vi "Polar (SubVI).vi"(11 "priorCoord":cluster{"x prior ":i32, "y prior":i32}) -> (2 "magnitude":dbl format="%0.2f", 3 "phase":dbl)   [LabVIEW 2011]
uses:
  <vilib>/Analysis/coordinate.llb/Angle Range (Degree).ctl
  <vilib>/Analysis/coordinate.llb/Angle Units.ctl
  <vilib>/Analysis/coordinate.llb/Wrap Angle (scalar).vi
  <vilib>/Analysis/NI_AAL_Angle.lvlib
  <vilib>/ptbypt/NI_PtbyPt.lvlib
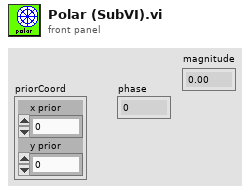
[diagram p1: front panel]
types:
  T1 = typedef "NI_AAL_Angle.lvlib/Angle Units.ctl" = i32
  T2 = typedef "NI_AAL_Angle.lvlib/Angle Range (Degree).ctl" = u16
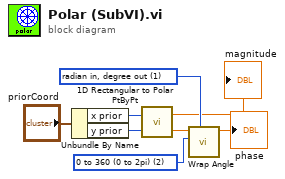
[diagram p0: block diagram]
diagram:
  w6 = T1 1 items=["radian in, radian out", "radian in, degree out", "degree in, degree out", "degree in, radian out"] ("angle units")
  w5 = T2 2 items=["none", "-180 to 180 (-pi to pi)", "0 to 360 (0 to 2pi)"] ("angle range")
  n1 = Unbundle By Name("priorCoord") -> ("x prior"=w2:i32, "y prior"=w3:i32)
  n2 = call <vilib>:"1D Rectangular to Polar PtByPt.vi"("y"=w3, "x"=w2) -> ("phase"=w4:dbl, "magnitude"=→"magnitude":dbl)
  n3 = call-poly <vilib>:"Wrap Angle.vi"("angle units"=w6, "angle range"=w5, "angle in"=w4) -> ("angle out"=→"phase":dbl)  [unwired: 7 in, 1 out]
